vi "VideoLoop.vi"   [LabVIEW 2015]
uses:
  <vilib>/Platform/TimedLoop/XDataNode/timing_clust.ctl
  <vilib>/Platform/TimedLoop/XDataNode/nitl_modes.ctl
  <vilib>/Platform/TimedLoop/XDataNode/wakeup.ctl
  <vilib>/Platform/TimedLoop/XDataNode/XDataNode.xnode
  <vilib>/Platform/TimedLoop/XDataNode/XDNodeRunTimeDep.lvlib
  Classes/CAlex2/CAlex2.lvclass
types:
  T1 = typedef "XDNodeRunTimeDep.lvlib/timing_clust.ctl" = cluster{"Expected End [f-1]":u64, "Actual End [f-1]":u64, "Finished Late? [f-1]":bool, "Expected End [i-1]":u64, "Actual End [i-1]":u64, "Finished Late? [i-1]":bool, "Expected Start [i]":u64, "Actual Start [i]":u64, "Expected Start [f]":u64, "Actual Start [f]":u64, "Source Name":string, "Structure Name":string, "Period":i64, "Deadline":i64, "Offset":i64, "Start":i64, "Priority":i32, "Timeout":i32, "Mode":T2, "Wakeup Reason":T3, "Error":errorcluster, "Source Type":string, "Secondary Source Type":string, "Global End Time":u64, "Global Start Time":u64, "Frame Duration":u64, "Iteration Duration":u64, "Assigned CPU":i32, "I/O Scan Engine Mode":u32}
  T2 = typedef "XDNodeRunTimeDep.lvlib/nitl_modes.ctl" = enum32{"No Change", "Process missed periods, maintain original phase", "Discard missed periods, maintain original phase", "Process missed periods, ignore original phase", "Discard missed periods, ignore original phase"}
  T3 = typedef "XDNodeRunTimeDep.lvlib/wakeup.ctl" = enum32{"Normal", "Aborted", "Asynchronous wakeup", "Timing source error", "Timed loop error", "Timeout"}
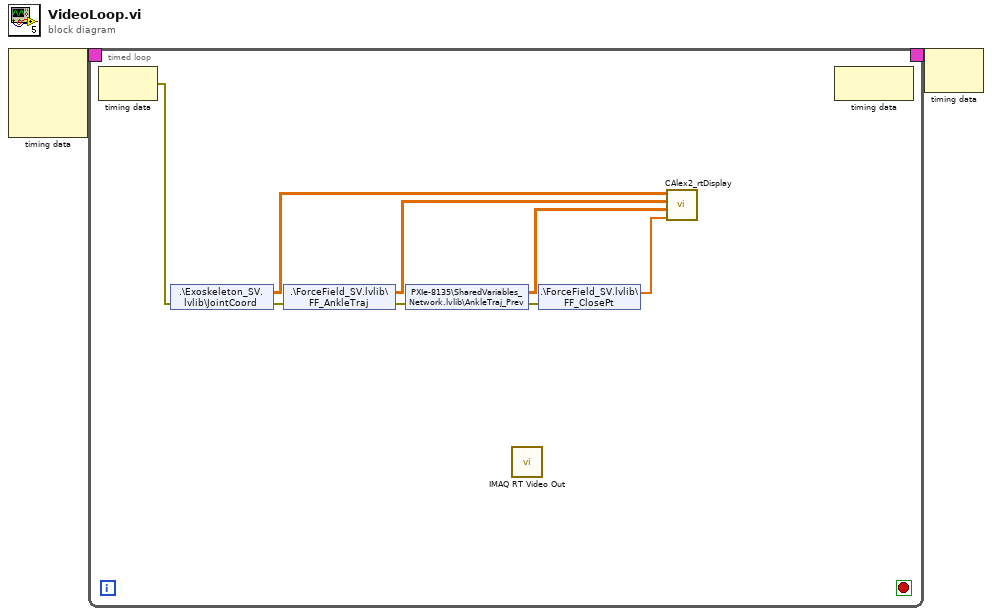
[diagram p0: block diagram]
diagram:
  n1 = node-c288() -> (w2:T1)  [unwired: 4 in]
  n2 = timed-loop {
    timing: w2 -> [_]
    timing-out: [_] -> w1
    stop <- _ stop-if-true
    n3 = node-c288() -> (w3:errorcluster)  [unwired: 1 in]
    n4 = shared-variable ".\\Exoskeleton_SV.lvlib\\JointCoord"(error in=w3) -> (w5:dbl[][], error out=w4:errorcluster)
    n5 = shared-variable ".\\ForceField_SV.lvlib\\FF_AnkleTraj"(error in=w4) -> (w8:dbl[][], error out=w7:errorcluster)
    n6 = shared-variable "PXIe-8135\\SharedVariables_Network.lvlib\\AnkleTraj_Prev"(error in=w7) -> (w9:dbl[][], error out=w6:errorcluster)
    n7 = call "IMAQ RT Video Out"() -> ()  [unwired: 10 in, 2 out]
    n8 = shared-variable ".\\ForceField_SV.lvlib\\FF_ClosePt"(error in=w6) -> (w10:dbl[])  [unwired: 1 out]
    n9 = call "CAlex2_rtDisplay.vi"("Cloest Pt"=w10, "PrevTraj"=w9, "TargetTraj"=w8, "JointLoc"=w5) -> ()  [unwired: 7 in, 1 out]
    n10 = node-c288() -> ()  [unwired: 1 in, 1 out]
  }
  n11 = node-c288(w1) -> ()  [unwired: 1 out]
